vi "MyPropertyClass_LV2009_GetAttributes.vi"(0 "reference in":refnum<class "MyPropertyClass_LV2009.lvclass">, 1 "return data? (T)":bool=TRUE, 5 "error in (no error)":errorcluster) -> (14 "reference out":refnum<class "MyPropertyClass_LV2009.lvclass">, 15 "attributes ref":T2, 16 "attributes":T1, 19 "error out":errorcluster)   [LabVIEW 2020, in "MyPropertyClass_LV2009.lvclass"]
doc: "Returns a reference and if wanted the actual data values of the attributes. This method is used by the subclasses to access parent attributes."
uses:
  MyPropertyClass_LV2009.lvclass
  ObjectAttributesRef.ctl
  protected/ObjectAttributes.ctl
  MyPropertyClass_LV2009.lvclass/MyPropertyClass_LV2009.ctl
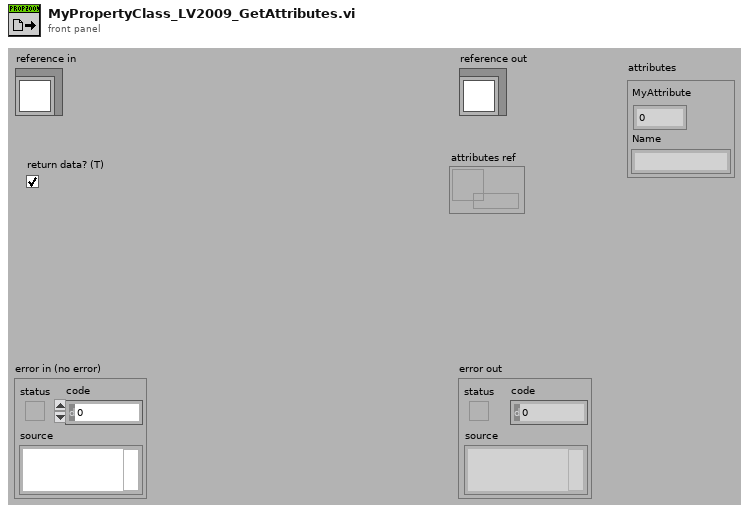
[diagram p1: front panel]
types:
  T1 = typedef "MyPropertyClass_LV2009.lvclass/ObjectAttributes.ctl" = cluster{"MyAttribute":dbl, "Name":string}
  T2 = typedef "MyPropertyClass_LV2009.lvclass/ObjectAttributesRef.ctl" = refnum<data-value>
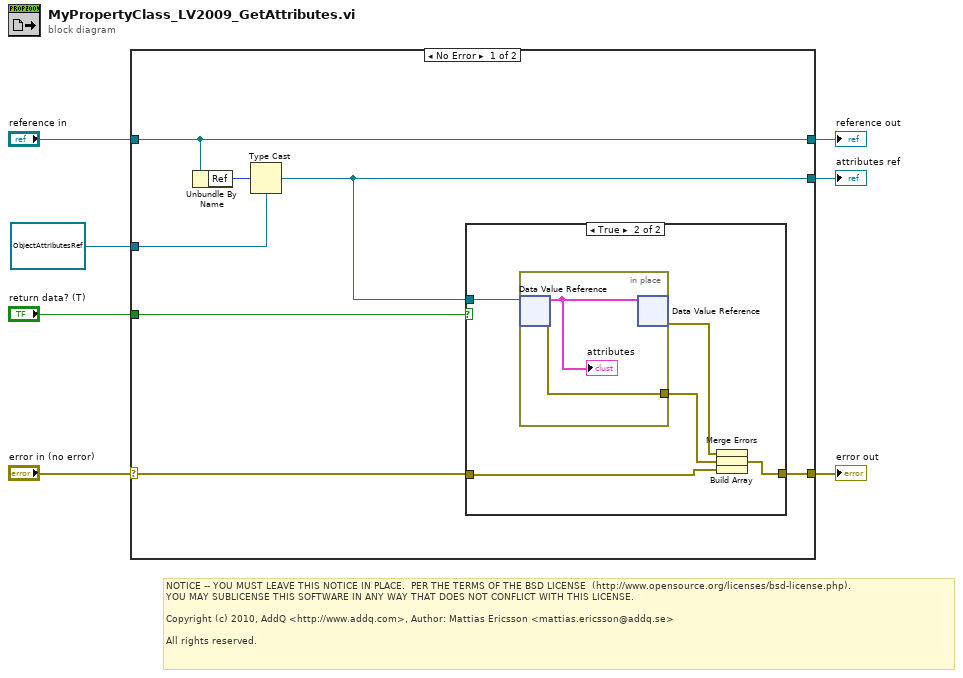
[diagram p0: block diagram]
diagram:
  # "NOTICE -- YOU MUST LEAVE THIS NOTICE IN PLACE.  PER THE TERMS OF THE BSD LICENSE  (http://www.opensource.org/licenses/bsd-license.php).\nYOU MAY SUBLICENSE THIS SOFTWARE IN ANY WAY THAT DOES NOT CONFLICT WITH THIS LICENSE.\n\nCopyright (c) 2010, AddQ <http://www.addq.com>, Author: Mattias Ericsson <mattias.ericsson@addq.se>\n\nAll rights reserved."
  n1 = case shown="No Error" "error in (no error)" {
    selector: "error in (no error)" -> [w12 w26]
    tunnel: [w11 w26] -> w6
    tunnel: [w14 w25] -> w4
    tunnel: "reference in" -> [w14 w25]
    tunnel: [w9 w24] -> w3
    tunnel: "return data? (T)" -> [w13 _]
    tunnel: T2 refnum ("attributes ref") -> [w8 w24]
    frame No Error {
      n2 = Unbundle By Name(w14) -> ("Ref"=w10:u32)
      n3 = Type Cast(type=w8, x=w10) -> (*(type *) &x=w9:T2)
      n4 = case shown="True" w13 {
        tunnel: w9 -> [_ w21]
        tunnel: w12 -> [w15 w20]
        tunnel: [w15 w17] -> w11
        frame False {
        }
        frame True {
          n5 = in-place {
            in-place-border: [w23] -> w19
            n6 = in-place-dvr #1(w21) -> (w22:T1, w23:errorcluster)
            "attributes" <- w22
            n7 = in-place-dvr #1(w22) -> (w18:errorcluster)  [unwired: 1 out]
          }
          n8 = Build Array(w18, w19, w20) -> (w16:errorcluster[])
          n9 = Merge Errors(w16) -> (w17:errorcluster)
        }
      }
    }
    frame Error {
    }
  }
  "error out" <- w6
  "reference out" <- w4
  "attributes ref" <- w3
